vi "Cleanup.vi"(8 "error in (no error)":errorcluster, 11 "PanelArray in":refnum<class "ArrayManager.lvclass">) -> (0 "error out":errorcluster)   [LabVIEW 2020, in "OOPanel.lvlib" / "ArrayManager.lvclass"]
uses:
  ArrayManager.lvclass
  ArrayManager.lvclass/ArrayManager.ctl
  Manager/Manager.lvclass
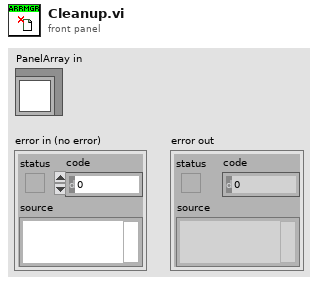
[diagram p1: front panel]
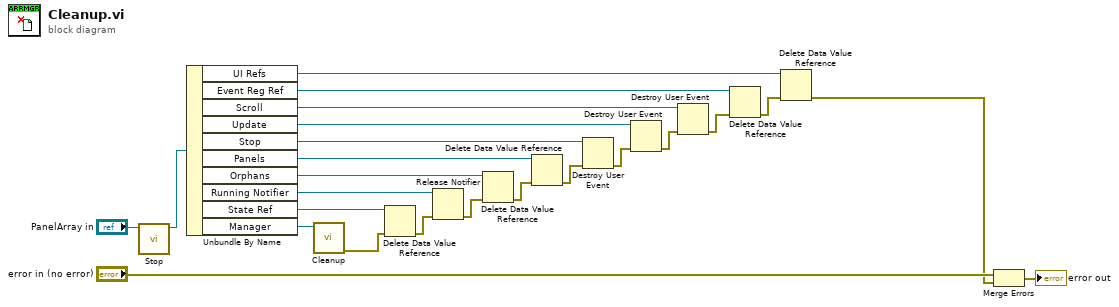
[diagram p0: block diagram]
diagram:
  n1 = call "Stop.vi"("ArrayManager in"="PanelArray in") -> ("ArrayManager out"=w20:refnum<class "ArrayManager.lvclass">)  [unwired: 9 in, 1 out]
  n2 = Unbundle By Name(w20) -> ("UI Refs"=w3:refnum<data-value>, "Event Reg Ref"=w5:refnum<data-value>, "Scroll"=w6:refnum<user-event>, "Update"=w9:refnum<user-event>, "Stop"=w11:refnum<user-event>, "Panels"=w14:refnum<data-value>, "Orphans"=w15:refnum<data-value>, "Running Notifier"=w17:refnum<notifier>, "State Ref"=w19:refnum<data-value>, "Manager"=w23:refnum<class "Manager.lvclass">)
  n3 = call "Cleanup.vi"("Manager in"=w23) -> ("error out"=w18:errorcluster)  [unwired: 8 in, 2 out]
  n4 = Delete Data Value Reference(data value reference=w19, error in=w18) -> (error out=w16:errorcluster)  [unwired: 1 out]
  n5 = Release Notifier(notifier=w17, error in (no error)=w16) -> (error out=w13:errorcluster)  [unwired: 1 in, 2 out]
  n6 = Delete Data Value Reference(data value reference=w15, error in=w13) -> (error out=w12:errorcluster)  [unwired: 1 out]
  n7 = Delete Data Value Reference(data value reference=w14, error in=w12) -> (error out=w10:errorcluster)  [unwired: 1 out]
  n8 = Destroy User Event(user event=w11, error in=w10) -> (error out=w8:errorcluster)
  n9 = Destroy User Event(user event=w9, error in=w8) -> (error out=w7:errorcluster)
  n10 = Destroy User Event(user event=w6, error in=w7) -> (error out=w4:errorcluster)
  n11 = Delete Data Value Reference(data value reference=w5, error in=w4) -> (error out=w2:errorcluster)  [unwired: 1 out]
  n12 = Delete Data Value Reference(data value reference=w3, error in=w2) -> (error out=w1:errorcluster)  [unwired: 1 out]
  n13 = Merge Errors("error in (no error)", w1) -> (→"error out":errorcluster)
